vi "GetCursorByName.vi"(10 "Name":string, 11 "IntensityGraph in":refnum<vi>) -> (0 "CursorInfo":T1, 2 "CursorRef":refnum<vi>, 3 "Found?":bool)   [LabVIEW 2017]
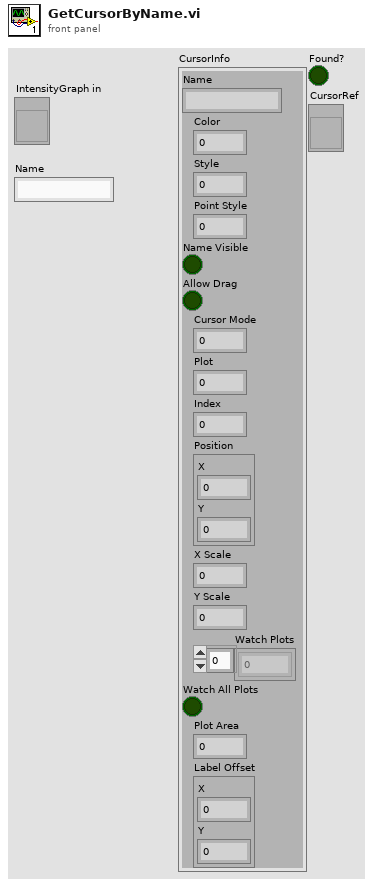
[diagram p1: front panel]
types:
  T1 = cluster{"Name":string, "Color":u32, "Style":u8, "Point Style":u8, "Name Visible":bool, "Allow Drag":bool, "Cursor Mode":u32, "Plot":i32, "Index":i32, "Position":cluster{"X":dbl, "Y":dbl}, "X Scale":u32, "Y Scale":u32, "Watch Plots":i32[], "Watch All Plots":bool, "Plot Area":i32, "Label Offset":cluster{"X":dbl, "Y":dbl}}
  T2 = typedef "LVCursorListTypeDef.ctl" = cluster{"Name":string, "Color":u32, "Style":u8, "Point Style":u8, "Name Visible":bool, "Allow Drag":bool, "Cursor Mode":u32, "Plot":i32, "Index":i32, "Position":cluster{"X":dbl, "Y":dbl}, "X Scale":u32, "Y Scale":u32, "Watch Plots":i32[], "Watch All Plots":bool, "Plot Area":i32, "Label Offset":cluster{"X":dbl, "Y":dbl}}[]
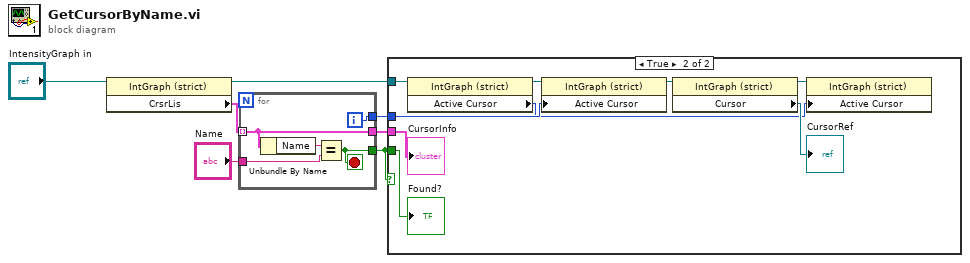
[diagram p0: block diagram]
diagram:
  n1 = property class="IntGraph (strict)"(reference="IntensityGraph in") -> (reference out=w1:refnum<vi>, "CrsrLis"=w6:T2)  [unwired: 1 in, 1 out]
  n2 = for {
    tunnel: w6 -> [w9] mode=indexing
    tunnel: "Name" -> [w11]
    tunnel: [w10] -> w2
    tunnel: [w9] -> w5
    tunnel: [w8] -> w3
    i -> [w8]
    stop <- w10 stop-if-true
    n3 = Unbundle By Name(w9) -> ("Name"=w12:string)
    n4 = Equal?(x=w12, y=w11) -> (x = y?=w10:bool)
  }
  n5 = case shown="True" w2 {
    tunnel: w5 -> [_ w21]
    tunnel: w2 -> [_ w20]
    tunnel: w3 -> [_ w19]
    tunnel: w1 -> [_ w13]
    frame False {
    }
    frame True {
      n6 = property class="IntGraph (strict)"(reference=w13) -> (reference out=w15:refnum<vi>, "Active Cursor"=w14:u32)  [unwired: 1 in, 1 out]
      n7 = property class="IntGraph (strict)"(reference=w15, "Active Cursor"=w19) -> (reference out=w18:refnum<vi>)  [unwired: 1 in, 1 out]
      n8 = property class="IntGraph (strict)"(reference=w18) -> (reference out=w17:refnum<vi>, "Cursor"=→"CursorRef":refnum<vi>)  [unwired: 1 in, 1 out]
      n9 = property class="IntGraph (strict)"(reference=w17, "Active Cursor"=w14) -> ()  [unwired: 1 in, 2 out]
      "CursorInfo" <- w21
      "Found?" <- w20
    }
  }
